vi "WFT AIO Channel Node Set.vi"(0 "WaveForms Session In":T1, 5 "idxChannel":i32, 7 "idxNode":i32, 9 "value":dbl, 11 "Error In":errorcluster) -> (4 "WaveForms Session Out":T1, 6 "ret":i32, 15 "Error Out":errorcluster)   [LabVIEW 2020, in "lv_waveforms_toolkit.lvlib"]
uses:
  lv_waveforms_toolkit.lvlib
  WFT Session.ctl
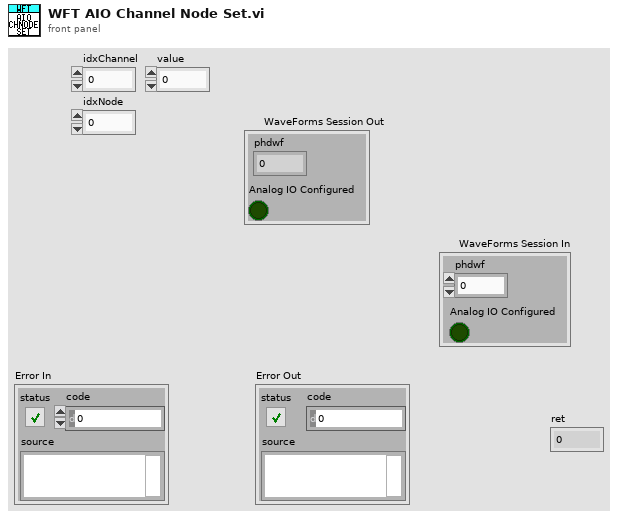
[diagram p1: front panel]
types:
  T1 = typedef "lv_waveforms_toolkit.lvlib/WFT Session.ctl" = cluster{"phdwf":i32, "Analog IO Configured":bool}
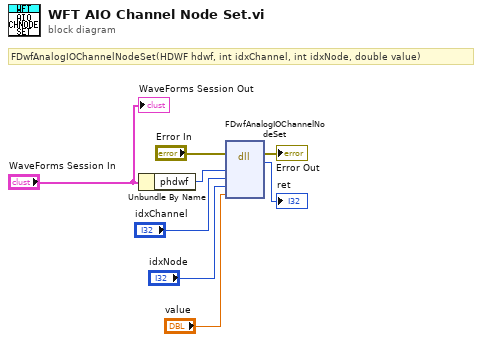
[diagram p0: block diagram]
diagram:
  # "FDwfAnalogIOChannelNodeSet(HDWF hdwf, int idxChannel, int idxNode, double value)"
  n1 = Unbundle By Name("WaveForms Session In") -> ("phdwf"=w4:i32)
  n2 = dll-call lib="dwf" fn="FDwfAnalogIOChannelNodeSet"(error in="Error In", "phdwf"=w4, "idxChannel"="idxChannel", "idxNode"="idxNode", "value"="value") -> (error out=→"Error Out":errorcluster, "return type"=→"ret":i32)  [unwired: 6 in, 1 out]
  "WaveForms Session Out" <- "WaveForms Session In"
